vi "LSX Get Stage SN.vi"(8 "error in (no error)":errorcluster, 9 "lMaxLen":i32, 10 "pcSN":string, 11 "lLSID":i32) -> (0 "error out":errorcluster, 2 "pcSN out":string, 3 "function return":i32)   [LabVIEW 2016, in "Tango_DLL.lvlib"]
doc: "TANGOAPI int TANGOCALL LSX_GetStageSN (int lLSID, char *pcSN, int lMaxLen);"
uses:
  Tango_DLL.lvlib
  2017/Microscope Control/Device Library/Stages/Marzhauser/SCAN IM 120 x 80/Tango DLL VIs/Tango_DLL.dll
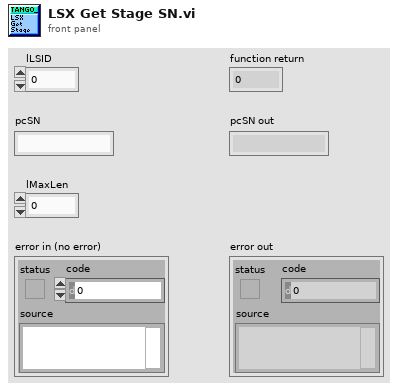
[diagram p1: front panel]
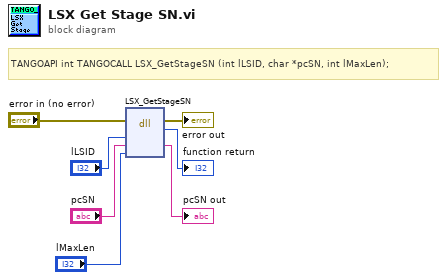
[diagram p0: block diagram]
diagram:
  # "TANGOAPI int TANGOCALL LSX_GetStageSN (int lLSID, char *pcSN, int lMaxLen);"
  n1 = dll-call lib="C:/Users/4PiSMS/Documents/Microscope Control/2017/Microscope Control/Device Library/Stages/Marzhauser/SCAN IM 120 x 80/Tango DLL VIs/Tango_DLL.*" fn="LSX_GetStageSN"(error in="error in (no error)", "lLSID"="lLSID", "pcSN"="pcSN", "lMaxLen"="lMaxLen") -> (error out=→"error out":errorcluster, →"function return":i32, "pcSN"=→"pcSN out":string)  [unwired: 4 in, 1 out]
